vi "getActualTemperature.vi"(8 "error in":T1) -> (0 "error out":T1, 3 "temperature":sgl format="%#_g K")   [LabVIEW 2016]
doc: "Retrives the current temperature in Kelvin."
uses:
  Controls/Error_Out.ctl
  Files_ASC500/DLL/ASC500_RemoteControlV27.dll
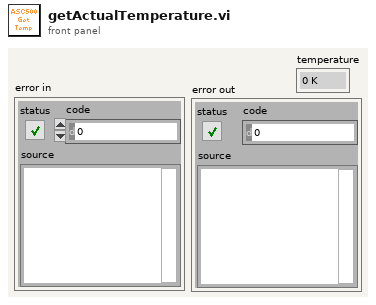
[diagram p1: front panel]
types:
  T1 = typedef "Error_Out.ctl" = errorcluster
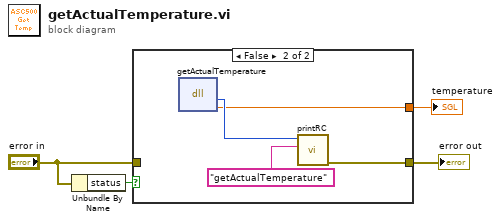
[diagram p0: block diagram]
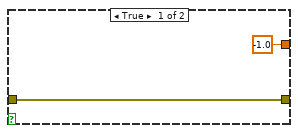
[diagram p2: hidden frame]
diagram:
  n1 = Unbundle By Name("error in") -> ("status"=w4:bool)
  n2 = case shown="False" w4 {
    tunnel: "error in" -> [w6 _]
    tunnel: [w6 w9] -> w2
    tunnel: [sgl -1.0 ("temperature") w7] -> w1
    frame True {
    }
    frame False {
      n3 = dll-call lib="G:/SCMOperations/Share/ELE/Produkt Information/ASC500/04 Remote Control/02 development versions/2018Nov06/Files_ASC500/DLL/ASC500_RemoteControlV27.dll" fn="getActualTemperature"() -> ("return type"=w8:i32, "temperature"=w7:sgl)  [unwired: 4 in, 2 out]
      n4 = call "printRC.vi"("additional information"="getActualTemperature", "RC"=w8) -> ("error out"=w9:T1)  [unwired: 9 in]
    }
  }
  "error out" <- w2
  "temperature" <- w1
